vi "test_psmc_v2.vi"() -> ()   [LabVIEW 2014]
uses:
  <vilib>/ptbypt/NI_PtbyPt.lvlib
panel:
  in  "Reset":bool
  out "f":dbl
  in  "pd":dbl
  out "reference vs actual":T1(graph)={"M1 desired speed"=-0.04979126824650304, "M1 position"=nan}
  in  "stop":bool
  # "This is desired position"
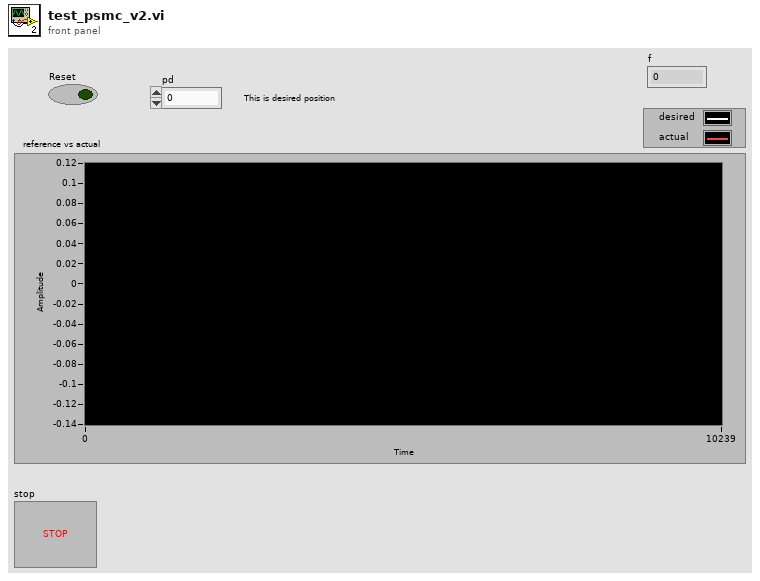
[diagram p1: front panel]
types:
  T1 = cluster{"M1 desired speed":dbl, "M1 position":dbl}
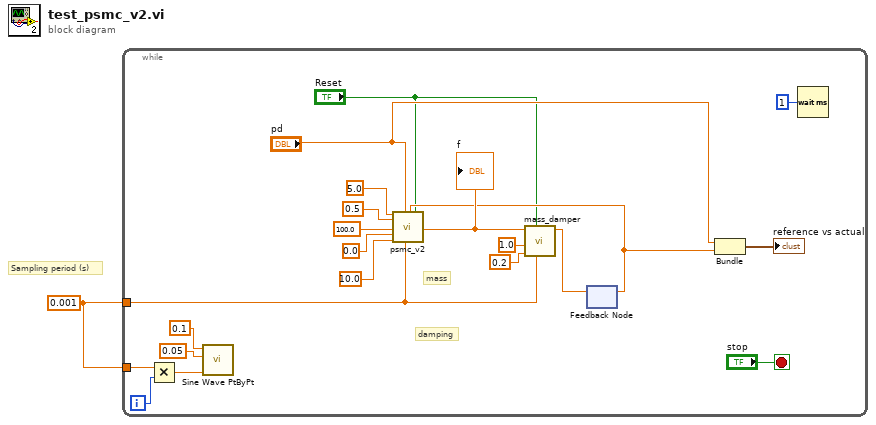
[diagram p0: block diagram]
diagram:
  w1 = 0.001 ("T")
  # "Sampling period (s)"
  n1 = while {
    tunnel: w1 -> [w17]
    tunnel: w1 -> [w12]
    i -> [w18]
    stop <- "stop" stop-if-true
    # "damping"
    # "mass"
    n2 = Multiply(x=w17, y=w18) -> (x*y=w21:dbl)
    n3 = call <vilib>:"Sine Wave PtByPt.vi"("time"=w21, "frequency"=0.05, "amplitude"=0.1) -> ()  [unwired: 1 in, 1 out]
    n4 = feedback #1() -> (w4:dbl)  [unwired: 1 in]
    n5 = call "psmc_v2.vi"("F"=5.0, "lambda"=0.5 ("H"), "Kp"=100.0 ("K"), "Ki"=0.0 ("L"), "Kd"=10.0 ("B"), "rd"="pd", "T"=w12, "r"=w4, "Reset?"="Reset") -> ("f"=w6:dbl)  [unwired: 10 in]
    "f" <- w6
    n6 = call "mass_damper.vi"("dt"=w12, "Reset"="Reset", "B"=0.2, "Mass"=1.0, "f(t)"=w6) -> ("x(t)"=w5:dbl)  [unwired: 4 in, 2 out]
    n7 = feedback-in #1(w5) -> ()
    n8 = Bundle("pd"="pd", "x(t)"=w4) -> (→"reference vs actual":cluster{"pd":dbl, "x(t)":dbl})  [unwired: 1 in]
    n9 = Wait (ms)(milliseconds to wait=u32 1) -> ()  [unwired: 1 out]
  }
